vi "Example 01.vi"() -> ()   [LabVIEW 2019, in "Grassfire Algorithm.lvclass"]
uses:
  Grassfire Algorithm.lvclass
  Direction--enum.ctl
  Solution Grid Cell--cluster.ctl
  Solution--picture ring.ctl
  Selection Grid Cell--array.ctl
  Selection--picture ring.ctl
panel:
  in  "Selection Grid":T1=[[{"Grid Value"=0}, {"Grid Value"=2}, {"Grid Value"=0}, {"Grid Value"=0}, {"Grid Value"=0}, {"Grid Value"=0}, {"Grid Value"=1}], [{"Grid Value"=0}, {"Grid Value"=0}, {"Grid Value"=0}, {"Grid Value"=0}, {"Grid Value"=0}, {"Grid Value"=0}, {"Grid Value"=0}], [{"Grid Value"=0}, {"Grid Value"=0}, {"Grid Value"=0}, {"Grid Value"=0}, {"Grid Value"=0}, {"Grid Value"=0}, {"Grid Value"=0}], [{"Grid Value"=0}, {"Grid Value"=1}, {"Grid Value"=1}, {"Grid Value"=1}, {"Grid Value"=1}, {"Grid Value"=1}, {"Grid Value"=0}], [{"Grid Value"=0}, {"Grid Value"=0}, {"Grid Value"=1}, {"Grid Value"=1}, {"Grid Value"=0}, {"Grid Value"=0}, {"Grid Value"=0}], [{"Grid Value"=0}, {"Grid Value"=0}, {"Grid Value"=0}, {"Grid Value"=0}, {"Grid Value"=0}, {"Grid Value"=3}, {"Grid Value"=0}], [{"Grid Value"=1}, {"Grid Value"=1}, {"Grid Value"=0}, {"Grid Value"=0}, {"Grid Value"=0}, {"Grid Value"=0}, {"Grid Value"=0}]]
  in  "Heading":T3=enum."Right"
  out "Solution":T4[][](array[typedef])
  out "Directions":T3[](array[typedef])
  out "Valid":bool
  # "VALID only if \n# Start = 1\n# End = 1"
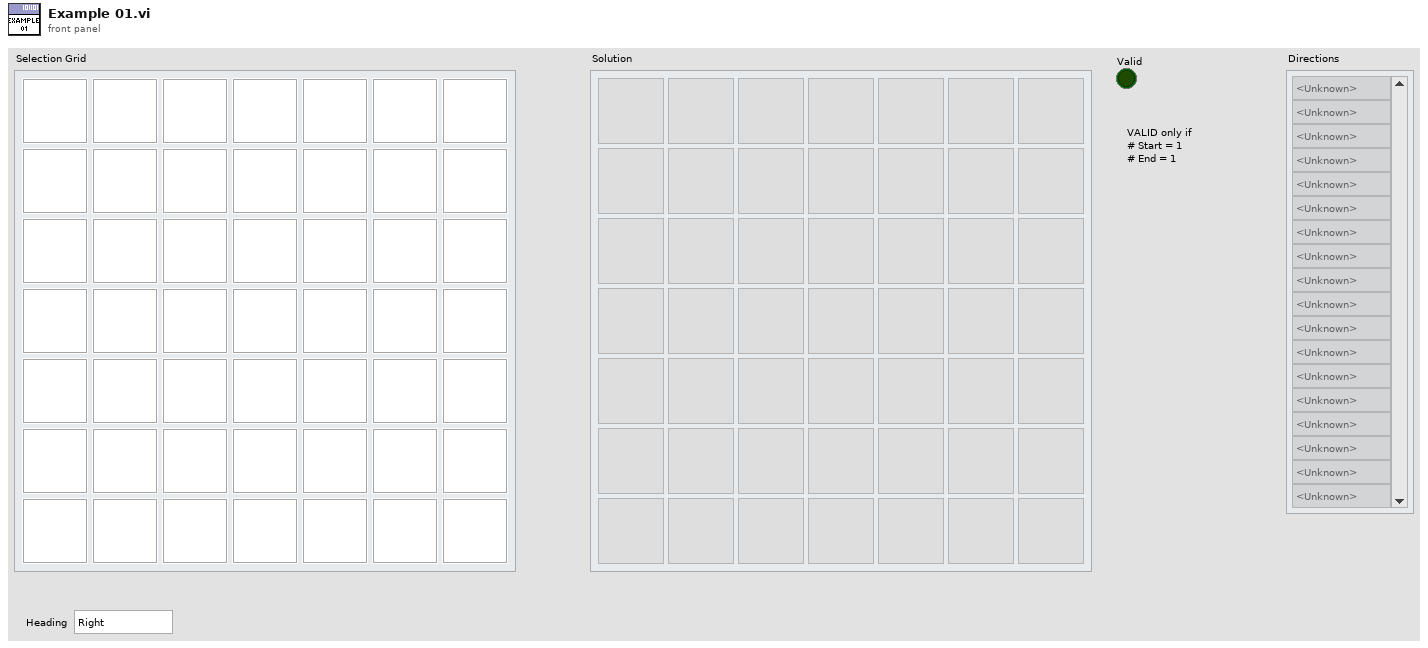
[diagram p1: front panel]
types:
  T1 = typedef "Grassfire Algorithm.lvclass/Selection Grid Cell--array.ctl" = cluster{"Grid Value":T2}[][]
  T2 = typedef "Grassfire Algorithm.lvclass/Selection--picture ring.ctl" = i64
  T3 = typedef "Grassfire Algorithm.lvclass/Direction--enum.ctl" = enum16{"<Unknown>", "Right", "Down", "Left", "Up"}
  T4 = typedef "Grassfire Algorithm.lvclass/Solution Grid Cell--cluster.ctl" = cluster{"Picture":T5, "Value":string}
  T5 = typedef "Grassfire Algorithm.lvclass/Solution--picture ring.ctl" = i64
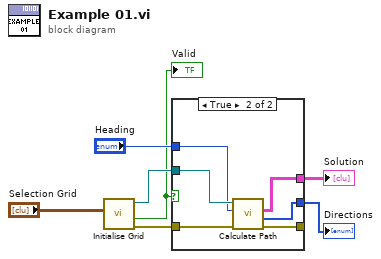
[diagram p0: block diagram]
diagram:
  n1 = call "Initialise Grid.vi"("Selection Grid"="Selection Grid") -> ("error out"=w6:errorcluster, "Valid"=w1:bool, "Grassfire Algorithm out"=w7:refnum<class "Grassfire Algorithm.lvclass">)  [unwired: 8 in]
  "Valid" <- w1
  n2 = case shown="True" w1 {
    tunnel: w7 -> [_ w14]
    tunnel: w6 -> [w8 w13]
    tunnel: [_ w12] -> w5
    tunnel: [_ w11] -> w3
    tunnel: "Heading" -> [_ w10]
    tunnel: [w8 w9] -> _
    frame False {
    }
    frame True {
      n3 = call-dynamic "Calculate Path.vi"("error in (no error)"=w13, "Direction Heading"=w10, "Module Data in"=w14) -> ("error out"=w9:errorcluster, "Directions"=w11:T3[], "Solution"=w12:T4[][])  [unwired: 5 in, 1 out]
    }
  }
  "Directions" <- w3
  "Solution" <- w5
